vi "ReadRoomEvents.vi"(8 "error in":errorcluster, 9 "columns":string[](array[string]), 10 "condition":string) -> (0 "error out":errorcluster, 2 "EventTimeArray":timestamp[](array[timestamp]), 3 "RoomArray":refnum<class "Room.lvclass">[](array[class]))   [LabVIEW 2015, in "DatabaseApi.lvlib"]
uses:
  DatabaseApi.lvlib
  LVClasses/Room/Room.lvclass
  TypeDef/Room/RoomTableDbTableName.ctl
  TypeDef/Room/RoomTableCluster.ctl
  <vilib>/addons/database/Connection.llb/DB Tools Open Connec (String).vi
  <vilib>/addons/database/_DB Variant To Data/Database Variant To Data.xnode
  <vilib>/addons/database/NI_Database_API.lvlib
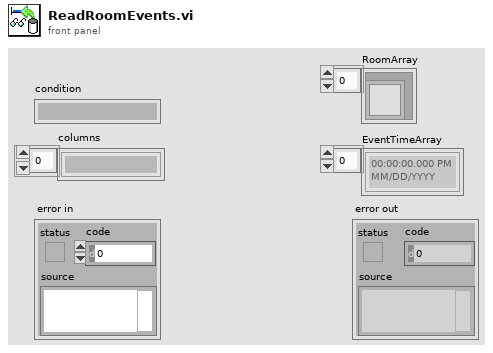
[diagram p1: front panel]
types:
  T1 = typedef "DatabaseApi.lvlib/RoomTableDbTableName.ctl" = string
  T2 = typedef "NI_Database_API.lvlib/Conn ObjectReference.ctl" = refnum<k1>
  T3 = typedef "DatabaseApi.lvlib/RoomTableCluster.ctl" = cluster{"Room Number":i32, "EventTime":timestamp, "Flag0":i32, "Flag1":i32, "Flag2":i32, "Flag3":i32, "FlagColors":string, "BedVacant":i32, "InRoomPersonnel":string}
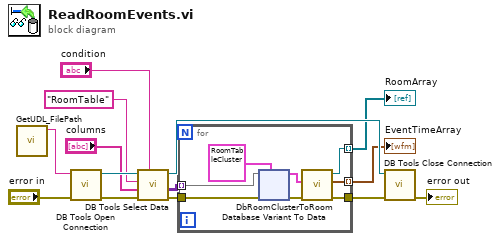
[diagram p0: block diagram]
diagram:
  n1 = call "GetUDL_FilePath.vi"() -> ("UDL file path"=w14:string)  [unwired: 11 in]
  n2 = call-poly <vilib>:"DB Tools Open Connection.vi"("error in (no error)"="error in", "connection information"=w14) -> ("error out"=w12:errorcluster, "connection reference"=w13:T2)  [unwired: 6 in]
  n3 = call <vilib>:"DB Tools Select Data.vi"("condition"="condition", "error in (no error)"=w12, "columns"="columns", "table"=T1 "RoomTable" ("RoomTableName"), "connection reference"=w13) -> ("error out"=w9:errorcluster, "data"=w7:variant[][], "connection reference out"=w6:T2)  [unwired: 1 in]
  n4 = for {
    tunnel: w9 -> [w22]
    tunnel: [w18] -> w8
    tunnel: w7 -> [w20] mode=indexing
    tunnel: [w16] -> w2 mode=indexing
    tunnel: [w15] -> w1 mode=indexing
    n5 = xnode "Database Variant To Data"("database variant"=w20, "error in (no error)"=w22, "type"=T3 {"Room Number"=0, "EventTime"=timestamp(0 s since 1904-01-01), "Flag0"=0, "Flag1"=0, "Flag2"=0, "Flag3"=0, "FlagColors"="", "BedVacant"=0, "InRoomPersonnel"=""} ("RoomTableCluster")) -> ("data"=w17:T3, "error out"=w21:errorcluster)
    n6 = call "DbRoomClusterToRoom.vi"("error in"=w21, "RoomTableCluster"=w17) -> ("error out"=w18:errorcluster, "EventTime"=w15:timestamp, "Room out"=w16:refnum<class "Room.lvclass">)  [unwired: 7 in]
  }
  "RoomArray" <- w2
  "EventTimeArray" <- w1
  n7 = call <vilib>:"DB Tools Close Connection.vi"("error in (no error)"=w8, "connection reference"=w6) -> ("error out"=→"error out":errorcluster)  [unwired: 5 in]
